vi "AtSpectrograph_acceptCommand_enable.vi"(8 "error in (no error)":errorcluster, 11 "command_enable_Ctl":T1) -> (0 "error out":errorcluster, 2 "function return":i32, 3 "command_enable_Ctl out":T1)   [LabVIEW 2016, in "SALLV_AtSpectrograph.lvlib"]
doc: "int AtSpectrograph_shm_acceptCommand_enableLV(AtSpectrograph_command_enableLV *command_enable_Ctl );"
uses:
  SALLV_AtSpectrograph.lvlib
  DataTypes/command_enable.ctl
  SALLV_AtSpectrograph.so
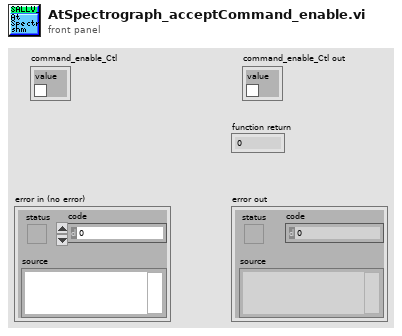
[diagram p1: front panel]
types:
  T1 = typedef "SALLV_AtSpectrograph.lvlib/command_enable.ctl" = cluster{"value":bool}
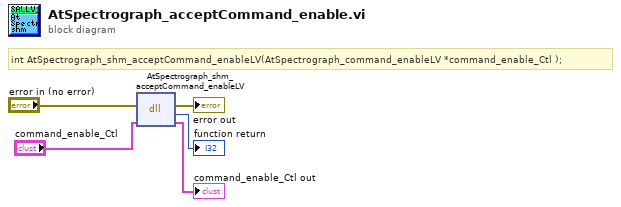
[diagram p0: block diagram]
diagram:
  # "int AtSpectrograph_shm_acceptCommand_enableLV(AtSpectrograph_command_enableLV *command_enable_Ctl );"
  n1 = dll-call lib="home/harini/tcs/temp/SALLV_AtSpectrograph/SALLV_AtSpectrograph.*" fn="AtSpectrograph_shm_acceptCommand_enableLV"(error in="error in (no error)", "command_enable_Ctl"="command_enable_Ctl") -> (error out=→"error out":errorcluster, →"function return":i32, "command_enable_Ctl"=→"command_enable_Ctl out":T1)  [unwired: 2 in, 1 out]
